vi "1PPS.vi"(1 "Read Index\nNumber":i32, 2 "UTC ts":u64, 3 "1PPS ts":u64, 4 "Action":T1(ring)) -> (0 "Array":u64[](array[numeric]))   [LabVIEW 2016]
panel:
  out "initialized array":u64[][](array[numeric])
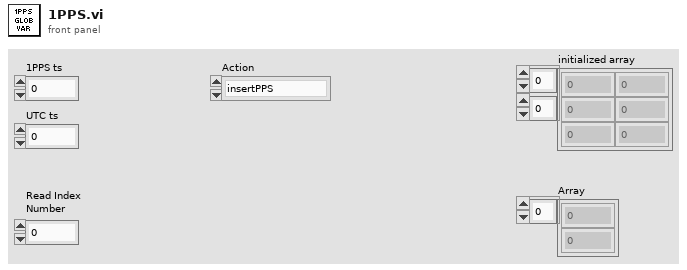
[diagram p1: front panel]
types:
  T1 = enum16{"insertPPS", "insertUTC", "read", "initiate"}
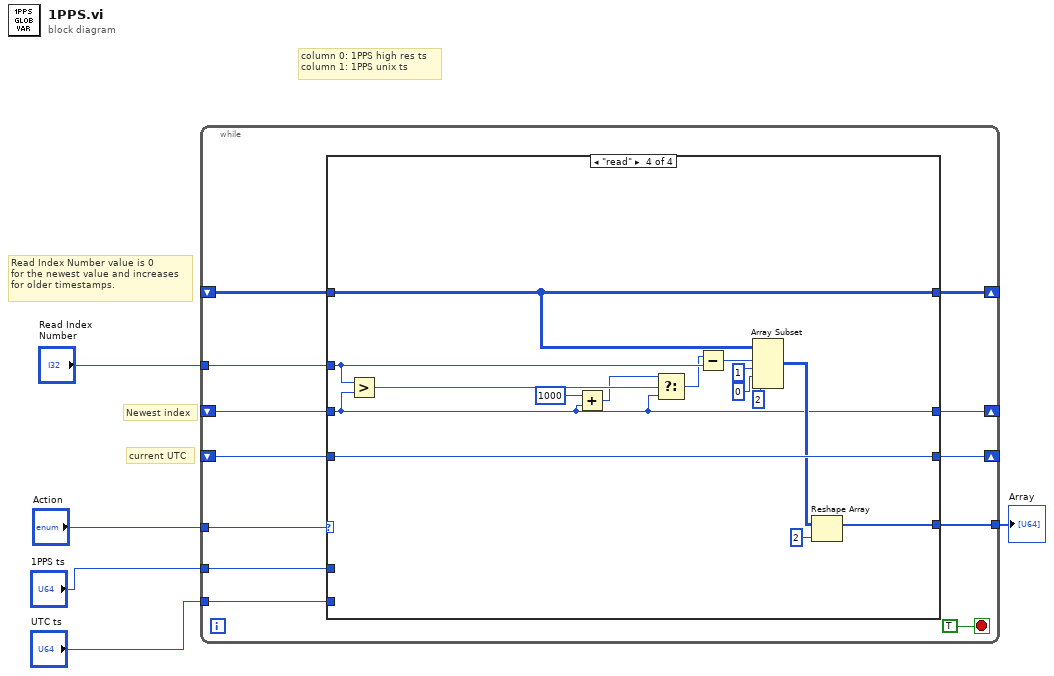
[diagram p0: block diagram]
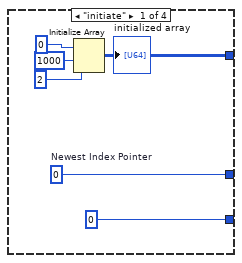
[diagram p2: hidden frame]
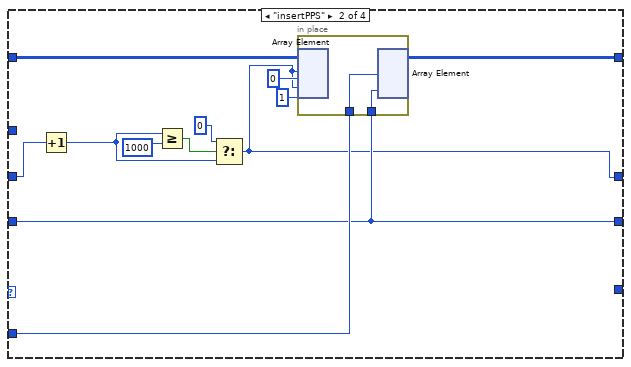
[diagram p3: hidden frame]
diagram:
  # "current UTC"
  # "Newest index"
  # "Read Index Number value is 0\nfor the newest value and increases\nfor older timestamps."
  # "column 0: 1PPS high res ts\ncolumn 1: 1PPS unix ts"
  n1 = while {
    tunnel: "Action" -> [w17]
    shift-right: [w13] -> _
    shift-left: _ -> [w15]
    shift-right: [w12] -> _
    shift-left: _ -> [w14]
    tunnel: "1PPS ts" -> [w11]
    tunnel: [w7] -> w1
    shift-right: [w9] -> _
    shift-left: _ -> [w10]
    tunnel: "UTC ts" -> [w8]
    tunnel: "Read Index\nNumber" -> [w6]
    stop <- TRUE stop-if-true
    n2 = case shown="\"read\"" w17 {
      tunnel: w15 -> [_ w28 w38 w54]
      tunnel: w14 -> [_ w30 w40 w45]
      tunnel: [w22 w24 w38 w54] -> w13
      tunnel: [w18 w25 w40 w45] -> w12
      tunnel: w11 -> [_ w32 _ _]
      tunnel: w10 -> [_ w31 _ w55]
      tunnel: [u32 0 ("1PPS ts") w31 w39 w55] -> w9
      tunnel: w8 -> [_ _ w39 _]
      tunnel: [_ _ _ w51] -> w7
      tunnel: w6 -> [_ _ _ w48]
      frame "initiate" {
        w18 = 0  # Newest Index Pointer
        n3 = Initialize Array(u64 0 ("element"), 1000 ("dimension size"), 2 ("dimension size")) -> (w22:u64[][])
        "initialized array" <- w22
      }
      frame "insertPPS" {
        n4 = Increment(x=w30) -> (x+1=w29:i32)
        n5 = Greater Or Equal?(x=w29, y=1000) -> (x >= y?=w34:bool)
        n6 = Select(t=0, s=w34, f=w29) -> (s? t:f=w25:i32)
        n7 = in-place {
          in-place-border: w32 -> [w37]
          in-place-border: w31 -> [w36]
          n8 = in-place-array #1(w28, w25, 0, w25, 1) -> ()  [unwired: 2 out]
          n9 = in-place-array #1(w37, w36) -> (w24:u64[][])  [unwired: 4 out]
        }
      }
      frame "insertUTC" {
      }
      frame "read" {
        n10 = Greater?(x=w48, y=w45) -> (0:w46:bool)
        n11 = Add(x=1000, y=w45) -> (x+y=w44:i32)
        n12 = Select(t=w44, s=w46, f=w45) -> (s? t:f=w47:i32)
        n13 = Subtract(x=w47, y=w48) -> (x-y=w49:i32)
        n14 = Array Subset(array=w54, index (row)=w49, length (row)=1 ("length"), index (col)=0 ("index"), length (col)=2 ("length")) -> (w53:u64[][])
        n15 = Reshape Array(w53, 2 ("dimension size")) -> (w51:u64[])
      }
    }
  }
  "Array" <- w1
